vi "Teleop.vi"(10 "Match Info":T1={"Autonomous Elapsed Seconds"=0.0, "TeleOp Elapsed Seconds"=0.0, "Disabled Elapsed Seconds"=0.0, "Visited Autonomous"=FALSE, "Visited TeleOp"=FALSE, "Visited Disabled"=FALSE, "Autonomous Settings"={"Autonomous Style"=enum."Independent", "VI Refnum"=refnum}}, 11 "Call Context":T2) -> ()   [LabVIEW 2016]
doc: "This VI is called for each TeleOp packet received from the DS where the robot is not disabled. It is often used to read from the joysticks and update I/O or to update setpoints for timed control loops. It should complete and return within 20 milliseconds or it may miss DS packets."
uses:
  <vilib>/Rock Robotics/WPI/DriverStation/WPI_DriverStationDerivedRobotMode.ctl
  <vilib>/Rock Robotics/WPI/DriverStation/WPI_DriverStationMatch Info.ctl
  <vilib>/Rock Robotics/WPI/Solenoid/WPI_SolenoidValue.ctl
  <vilib>/Rock Robotics/WPI/Utilities/WPI_GetSetVariantRefNum.vi
  <vilib>/Rock Robotics/WPI/Solenoid/WPI_SolenoidSetEnum.vi
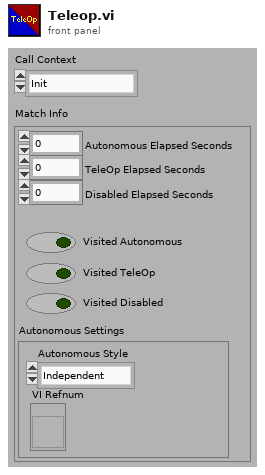
[diagram p1: front panel]
types:
  T1 = typedef "WPI_DriverStationMatch Info.ctl" = cluster{"Autonomous Elapsed Seconds":dbl, "TeleOp Elapsed Seconds":dbl, "Disabled Elapsed Seconds":dbl, "Visited Autonomous":bool, "Visited TeleOp":bool, "Visited Disabled":bool, "Autonomous Settings":cluster{"Autonomous Style":enum16{"Iterative", "Independent"}, "VI Refnum":refnum<vi>}}
  T2 = typedef "WPI_DriverStationDerivedRobotMode.ctl" = enum16{"Init", "Execute", "Stop"}
  T3 = enum16{"Initialization", "Rotate the Arm & Open Grabber", "Bring Arm Down", "Grab the Gear & Bring Back Up", "Rotate the Gear & Ready to Launch"}
  T4 = typedef "WPI_JoystickDevRef.ctl" = cluster{"Device":T5}
  T5 = typedef "WPI_JoystickDeviceEnum.ctl" = enum16{"USB 0", "USB 1", "USB 2", "USB 3", "USB 4", "USB 5"}
  T6 = cluster{"Buttons[0]":bool, "Buttons[1]":bool, "Buttons[2]":bool, "Buttons[3]":bool, "Buttons[4]":bool, "Buttons[5]":bool, "Buttons[6]":bool, "Buttons[7]":bool, "Buttons[8]":bool}
  T7 = cluster{"Axes[0]":dbl, "Axes[1]":dbl, "Axes[2]":dbl, "Axes[3]":dbl, "Axes[4]":dbl, "Axes[5]":dbl, "Axes[6]":dbl, "Axes[7]":dbl, "Axes[8]":dbl}
  T8 = typedef "WPI_SolenoidValue.ctl" = enum16{"Off", "On", "Forward", "Reverse"}
  T9 = typedef "WPI_SolenoidDevRef.ctl" = cluster{"DevStatus":errorcluster, "Pneumatics Control Module":u8, "Forward Solenoid Channel":T10, "Reverse Solenoid Channel":T10}
  T10 = typedef "WPI_SolenoidChannel.ctl" = enum8{"Solenoid 0", "Solenoid 1", "Solenoid 2", "Solenoid 3", "Solenoid 4", "Solenoid 5", "Solenoid 6", "Solenoid 7", "Invalid"}
  T11 = typedef "WPI_MotorControlDeviceRef.ctl" = cluster{"DeviceStatus":errorcluster, "Type":T12, "PWM":cluster{"PWM Channel":T13, "DeadBand":T14}, "CAN":cluster{"Device Number":u8, "SetOutput VI Ref":variant, "GetOutput VI Ref":variant, "Enable VI Ref":variant, "Disable VI Ref":variant, "Data":variant}, "Invert":bool}
  T12 = typedef "WPI_MotorControlType.ctl" = enum16{"PWM", "CAN"}
  T13 = typedef "FPGA_DIOPWMChannel.ctl" = enum8{"PWM 0", "PWM 1", "PWM 2", "PWM 3", "PWM 4", "PWM 5", "PWM 6", "PWM 7", "PWM 8", "PWM 9", "PWM MXP 0", "PWM MXP 1", "PWM MXP 2", "PWM MXP 3", "PWM MXP 4", "PWM MXP 5", "PWM MXP 6", "PWM MXP 7", "PWM MXP 8", "PWM MXP 9", "Invalid"}
  T14 = typedef "WPI_PWMDeadband.ctl" = cluster{"Name":string, "maxPositivePwm":i32, "minPositivePwm":i32, "centerPwm":i32, "maxNegativePwm":i32, "minNegativePwm":i32, "angularRange":u16}
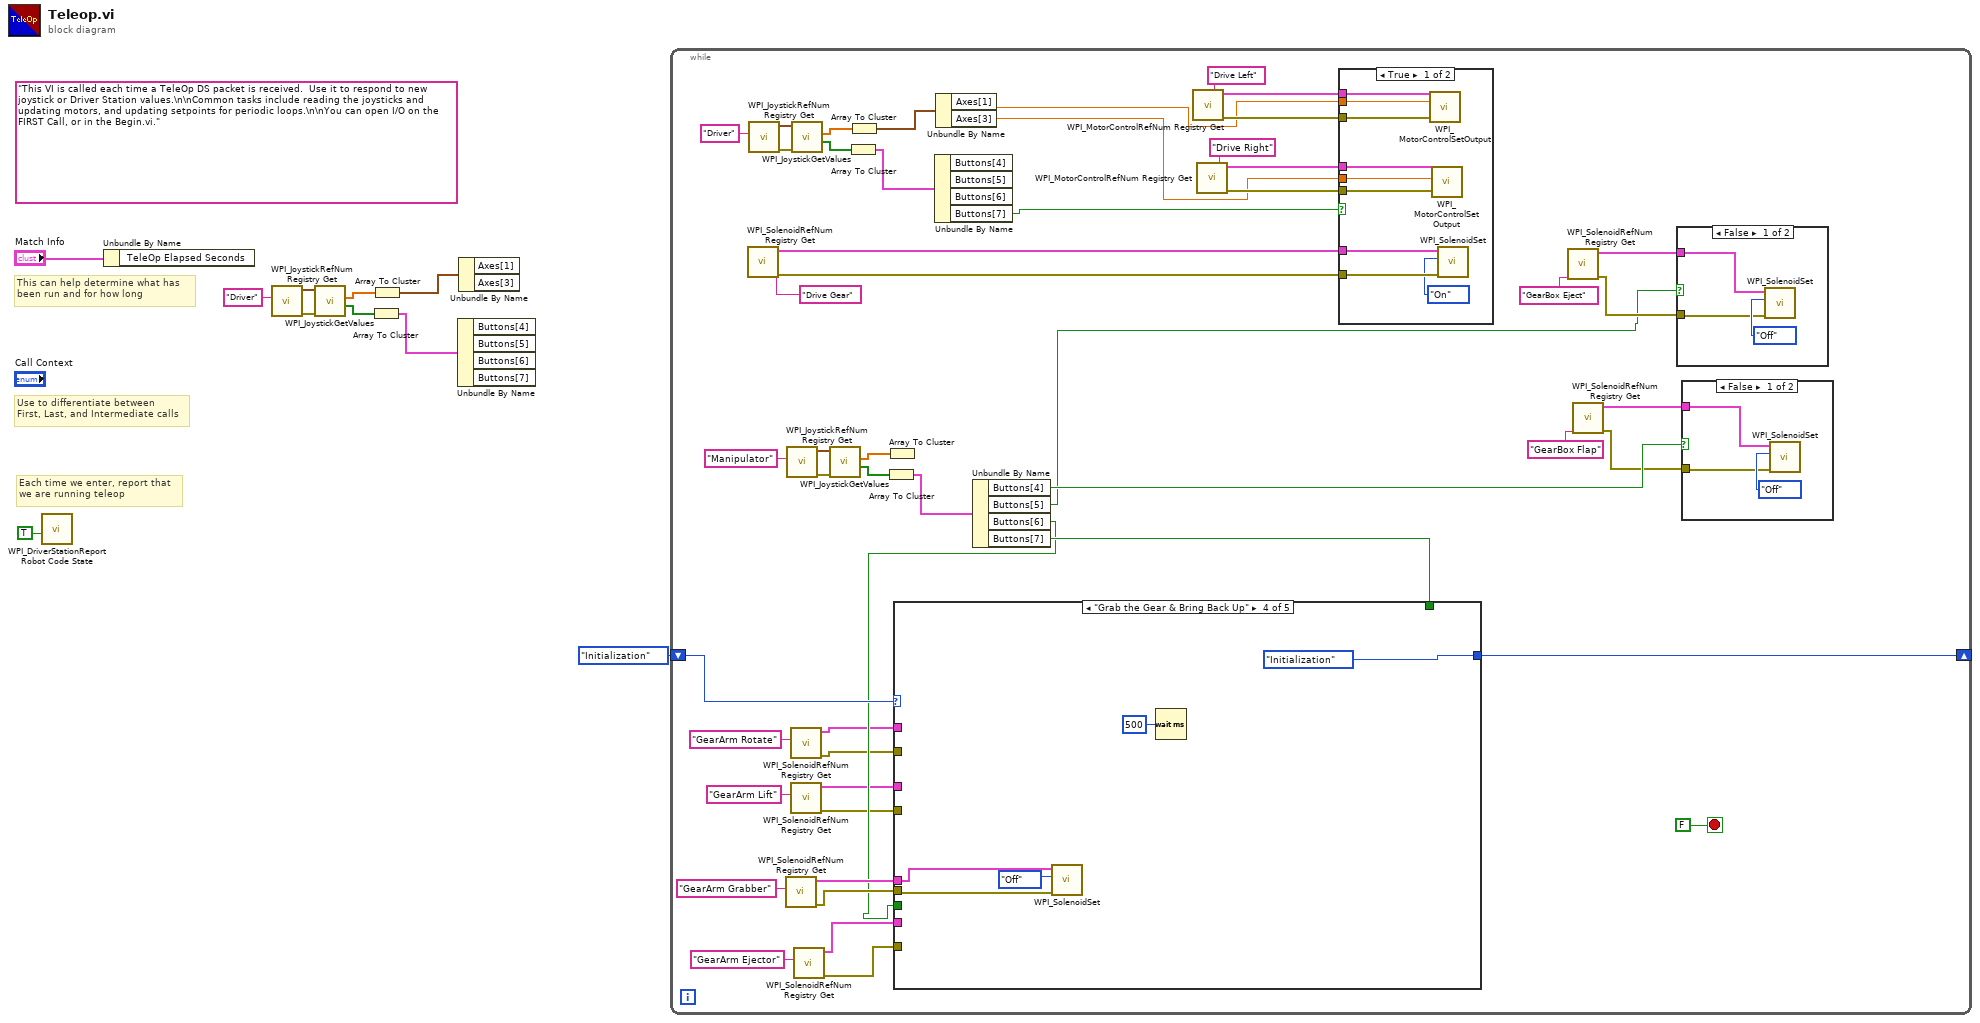
[diagram p0: block diagram]
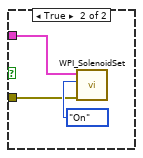
[diagram p2: hidden frame]
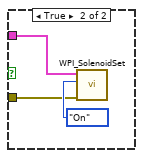
[diagram p3: hidden frame]
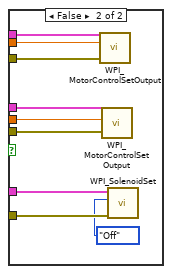
[diagram p4: hidden frame]
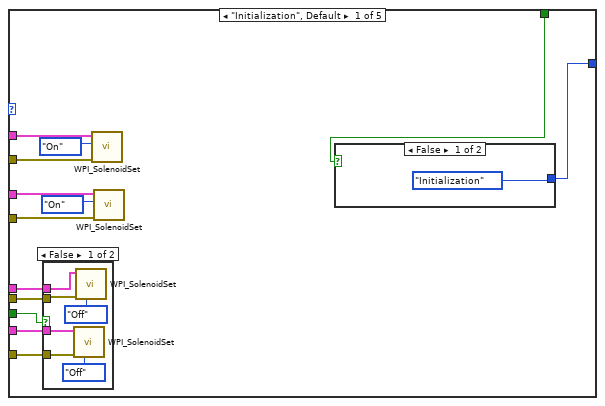
[diagram p5: hidden frame]
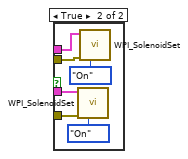
[diagram p6: hidden frame]
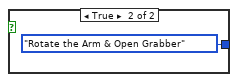
[diagram p7: hidden frame]
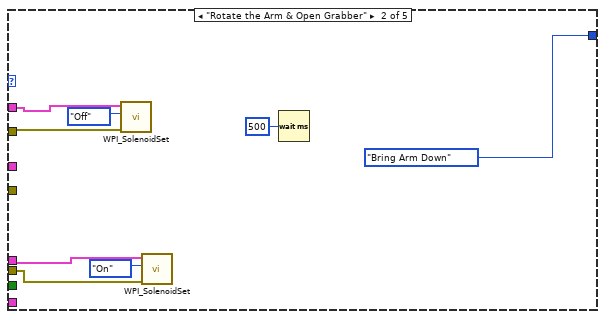
[diagram p8: hidden frame]
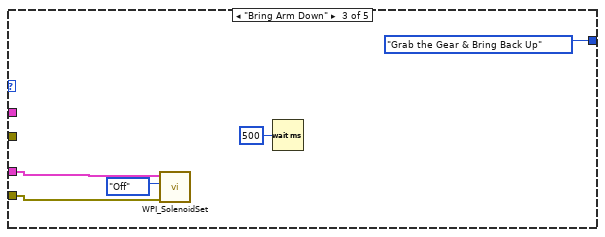
[diagram p9: hidden frame]
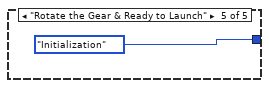
[diagram p10: hidden frame]
diagram:
  (unwired) "This VI is called each time a TeleOp DS packet is received.  Use it to respond to new joystick or Driver Station values.\n\nCommon tasks include reading the joysticks and updating motors, and updating setpoints for periodic loops.\n\nYou can open I/O on the FIRST Call, or in the Begin.vi."
  # "Each time we enter, report that\nwe are running teleop"
  # "Use to differentiate between\nFirst, Last, and Intermediate calls"
  # "This can help determine what has\nbeen run and for how long"
  n1 = call <vilib>:"WPI_DriverStationReport Robot Code State.vi"("TeleOp"=TRUE ("Autonomous")) -> ()  [unwired: 10 in, 1 out]
  n2 = Unbundle By Name("Match Info") -> ()  [unwired: 1 out]
  n3 = call <vilib>:"WPI_JoystickRefNum Registry Get.vi"("refnum name"="Driver") -> ("error out"=w7:errorcluster, "JoystickDevRef"=w6:T4)  [unwired: 9 in]
  n4 = call <vilib>:"WPI_JoystickGetValues.vi"("error in (no error)"=w7, "JoystickDevRef"=w6) -> ("Buttons"=w5:bool[], "Axes"=w4:dbl[])  [unwired: 5 in, 3 out]
  n5 = Array To Cluster(array=w5) -> (cluster=w2:T6)
  n6 = Array To Cluster(array=w4) -> (cluster=w3:T7)
  n7 = Unbundle By Name(w2) -> ()  [unwired: 4 out]
  n8 = Unbundle By Name(w3) -> ()  [unwired: 2 out]
  n9 = while {
    shift-right: [w34] -> _
    shift-left: T3."Initialization" -> [w54]
    stop <- FALSE stop-if-true
    n10 = call <vilib>:"WPI_SolenoidRefNum Registry Get.vi"("refnum name"="Drive Gear") -> ("error out"=w37:errorcluster, "SolenoidDevRef"=w38:T9)  [unwired: 9 in]
    n11 = call <vilib>:"WPI_JoystickRefNum Registry Get.vi"("refnum name"="Driver") -> ("error out"=w52:errorcluster, "JoystickDevRef"=w51:T4)  [unwired: 9 in]
    n12 = call <vilib>:"WPI_SolenoidRefNum Registry Get.vi"("refnum name"="GearArm Grabber") -> ("error out"=w18:errorcluster, "SolenoidDevRef"=w19:T9)  [unwired: 9 in]
    n13 = call <vilib>:"WPI_JoystickRefNum Registry Get.vi"("refnum name"="Manipulator") -> ("error out"=w56:errorcluster, "JoystickDevRef"=w57:T4)  [unwired: 9 in]
    n14 = call <vilib>:"WPI_SolenoidRefNum Registry Get.vi"("refnum name"="GearArm Rotate") -> ("error out"=w11:errorcluster, "SolenoidDevRef"=w12:T9)  [unwired: 9 in]
    n15 = call <vilib>:"WPI_SolenoidRefNum Registry Get.vi"("refnum name"="GearArm Lift") -> ("error out"=w14:errorcluster, "SolenoidDevRef"=w15:T9)  [unwired: 9 in]
    n16 = call <vilib>:"WPI_JoystickGetValues.vi"("error in (no error)"=w52, "JoystickDevRef"=w51) -> ("Buttons"=w50:bool[], "Axes"=w49:dbl[])  [unwired: 5 in, 3 out]
    n17 = call <vilib>:"WPI_SolenoidRefNum Registry Get.vi"("refnum name"="GearArm Ejector") -> ("error out"=w21:errorcluster, "SolenoidDevRef"=w22:T9)  [unwired: 9 in]
    n18 = call <vilib>:"WPI_JoystickGetValues.vi"("error in (no error)"=w56, "JoystickDevRef"=w57) -> ("Buttons"=w58:bool[], "Axes"=w59:dbl[])  [unwired: 5 in, 3 out]
    n19 = Array To Cluster(array=w50) -> (cluster=w47:T6)
    n20 = Array To Cluster(array=w49) -> (cluster=w48:T7)
    n21 = Array To Cluster(array=w58) -> (cluster=w60:T6)
    n22 = Array To Cluster(array=w59) -> ()  [unwired: 1 out]
    n23 = Unbundle By Name(w47) -> ("Buttons[7]"=w35:bool)  [unwired: 3 out]
    n24 = Unbundle By Name(w48) -> ("Axes[1]"=w42:dbl, "Axes[3]"=w41:dbl)
    n25 = Unbundle By Name(w60) -> ("Buttons[4]"=w30:bool, "Buttons[5]"=w24:bool, "Buttons[6]"=w17:bool, "Buttons[7]"=w32:bool)
    n26 = case shown="\"Grab the Gear & Bring Back Up\"" w54 {
      tunnel: [w103 T3."Bring Arm Down" T3."Grab the Gear & Bring Back Up" T3."Initialization" T3."Initialization"] -> w34
      tunnel: w32 -> [w102 _ _ _ _]
      tunnel: w22 -> [w101 _ _ _ _]
      tunnel: w21 -> [w100 _ _ _ _]
      tunnel: w19 -> [w99 w119 _ w132 _]
      tunnel: w18 -> [w98 w120 _ w133 _]
      tunnel: w17 -> [w97 _ _ _ _]
      tunnel: w15 -> [w96 _ w128 _ _]
      tunnel: w14 -> [w95 _ w127 _ _]
      tunnel: w12 -> [w92 w123 _ _ _]
      tunnel: w11 -> [w91 w122 _ _ _]
      frame "Initialization", Default {
        n27 = case shown="False" w97 {
          tunnel: w101 -> [w105 w114]
          tunnel: w100 -> [w104 w113]
          tunnel: w99 -> [w107 w111]
          tunnel: w98 -> [w106 w110]
          frame False {
            n28 = call-poly <vilib>:"WPI_SolenoidSet.vi"("error in (no error)"=w104, "Value"=WPI_SolenoidValue."Off", "SolenoidDevRef"=w105) -> ()  [unwired: 7 in, 2 out]
            n29 = call-poly <vilib>:"WPI_SolenoidSet.vi"("error in (no error)"=w106, "Value"=WPI_SolenoidValue."Off", "SolenoidDevRef"=w107) -> ()  [unwired: 7 in, 2 out]
          }
          frame True {
            n30 = call-poly <vilib>:"WPI_SolenoidSet.vi"("error in (no error)"=w113, "Value"=WPI_SolenoidValue."On", "SolenoidDevRef"=w114) -> ()  [unwired: 7 in, 2 out]
            n31 = call-poly <vilib>:"WPI_SolenoidSet.vi"("error in (no error)"=w110, "Value"=WPI_SolenoidValue."On", "SolenoidDevRef"=w111) -> ()  [unwired: 7 in, 2 out]
          }
        }
        n32 = call-poly <vilib>:"WPI_SolenoidSet.vi"("error in (no error)"=w91, "Value"=WPI_SolenoidValue."On", "SolenoidDevRef"=w92) -> ()  [unwired: 7 in, 2 out]
        n33 = call-poly <vilib>:"WPI_SolenoidSet.vi"("error in (no error)"=w95, "Value"=WPI_SolenoidValue."On", "SolenoidDevRef"=w96) -> ()  [unwired: 7 in, 2 out]
        n34 = case shown="False" w102 {
          tunnel: [T3."Initialization" T3."Rotate the Arm & Open Grabber"] -> w103
          frame False {
          }
          frame True {
          }
        }
      }
      frame "Rotate the Arm & Open Grabber" {
        n35 = call-poly <vilib>:"WPI_SolenoidSet.vi"("error in (no error)"=w122, "Value"=WPI_SolenoidValue."Off", "SolenoidDevRef"=w123) -> ()  [unwired: 7 in, 2 out]
        n36 = call-poly <vilib>:"WPI_SolenoidSet.vi"("error in (no error)"=w120, "Value"=WPI_SolenoidValue."On", "SolenoidDevRef"=w119) -> ()  [unwired: 7 in, 2 out]
        n37 = Wait (ms)(milliseconds to wait=u32 500) -> ()  [unwired: 1 out]
      }
      frame "Bring Arm Down" {
        n38 = call-poly <vilib>:"WPI_SolenoidSet.vi"("error in (no error)"=w127, "Value"=WPI_SolenoidValue."Off", "SolenoidDevRef"=w128) -> ()  [unwired: 7 in, 2 out]
        n39 = Wait (ms)(milliseconds to wait=u32 500) -> ()  [unwired: 1 out]
      }
      frame "Grab the Gear & Bring Back Up" {
        n40 = call-poly <vilib>:"WPI_SolenoidSet.vi"("error in (no error)"=w133, "Value"=WPI_SolenoidValue."Off", "SolenoidDevRef"=w132) -> ()  [unwired: 7 in, 2 out]
        n41 = Wait (ms)(milliseconds to wait=u32 500) -> ()  [unwired: 1 out]
      }
      frame "Rotate the Gear & Ready to Launch" {
      }
    }
    n42 = call <vilib>:"WPI_MotorControlRefNum Registry Get.vi"("refnum name"="Drive Left") -> ("error out"=w45:errorcluster, "MotorControlDevRef"=w46:T11)  [unwired: 9 in]
    n43 = call <vilib>:"WPI_MotorControlRefNum Registry Get.vi"("refnum name"="Drive Right") -> ("error out"=w43:errorcluster, "MotorControlDevRef"=w44:T11)  [unwired: 9 in]
    n44 = case shown="True" w35 {
      tunnel: w46 -> [w81 w90]
      tunnel: w45 -> [w80 w89]
      tunnel: w44 -> [w79 w88]
      tunnel: w43 -> [w78 w87]
      tunnel: w42 -> [w77 w86]
      tunnel: w41 -> [w76 w85]
      tunnel: w38 -> [w75 w84]
      tunnel: w37 -> [w74 w83]
      frame True {
        n45 = call <vilib>:"WPI_MotorControlSetOutput.vi"("error in (no error)"=w80, "Output"=w77, "MotorControlDevRef"=w81) -> ()  [unwired: 6 in, 3 out]
        n46 = call <vilib>:"WPI_MotorControlSetOutput.vi"("error in (no error)"=w78, "Output"=w76, "MotorControlDevRef"=w79) -> ()  [unwired: 6 in, 3 out]
        n47 = call-poly <vilib>:"WPI_SolenoidSet.vi"("error in (no error)"=w74, "Value"=WPI_SolenoidValue."On", "SolenoidDevRef"=w75) -> ()  [unwired: 7 in, 2 out]
      }
      frame False {
        n48 = call <vilib>:"WPI_MotorControlSetOutput.vi"("error in (no error)"=w89, "Output"=w86, "MotorControlDevRef"=w90) -> ()  [unwired: 6 in, 3 out]
        n49 = call <vilib>:"WPI_MotorControlSetOutput.vi"("error in (no error)"=w87, "Output"=w85, "MotorControlDevRef"=w88) -> ()  [unwired: 6 in, 3 out]
        n50 = call-poly <vilib>:"WPI_SolenoidSet.vi"("error in (no error)"=w83, "Value"=WPI_SolenoidValue."Off", "SolenoidDevRef"=w84) -> ()  [unwired: 7 in, 2 out]
      }
    }
    n51 = call <vilib>:"WPI_SolenoidRefNum Registry Get.vi"("refnum name"="GearBox Eject") -> ("error out"=w25:errorcluster, "SolenoidDevRef"=w26:T9)  [unwired: 9 in]
    n52 = call <vilib>:"WPI_SolenoidRefNum Registry Get.vi"("refnum name"="GearBox Flap") -> ("error out"=w28:errorcluster, "SolenoidDevRef"=w29:T9)  [unwired: 9 in]
    n53 = case shown="False" w24 {
      tunnel: w26 -> [w62 w65]
      tunnel: w25 -> [w61 w64]
      frame False {
        n54 = call-poly <vilib>:"WPI_SolenoidSet.vi"("error in (no error)"=w61, "Value"=WPI_SolenoidValue."Off", "SolenoidDevRef"=w62) -> ()  [unwired: 7 in, 2 out]
      }
      frame True {
        n55 = call-poly <vilib>:"WPI_SolenoidSet.vi"("error in (no error)"=w64, "Value"=WPI_SolenoidValue."On", "SolenoidDevRef"=w65) -> ()  [unwired: 7 in, 2 out]
      }
    }
    n56 = case shown="False" w30 {
      tunnel: w29 -> [w68 w71]
      tunnel: w28 -> [w67 w70]
      frame False {
        n57 = call-poly <vilib>:"WPI_SolenoidSet.vi"("error in (no error)"=w67, "Value"=WPI_SolenoidValue."Off", "SolenoidDevRef"=w68) -> ()  [unwired: 7 in, 2 out]
      }
      frame True {
        n58 = call-poly <vilib>:"WPI_SolenoidSet.vi"("error in (no error)"=w70, "Value"=WPI_SolenoidValue."On", "SolenoidDevRef"=w71) -> ()  [unwired: 7 in, 2 out]
      }
    }
  }
